vi "Pre Post Object File Path.vi"(6 "Post":string, 9 "Pre":string, 10 "Rename Library File Path":path) -> (1 "Post Object File Path":path, 2 "Pre Object File Path":path)   [LabVIEW 2025, in "_Rename.lvlib" / "_Rename.lvclass"]
uses:
  _Rename.lvclass
  _Rename.lvclass/_Rename.ctl
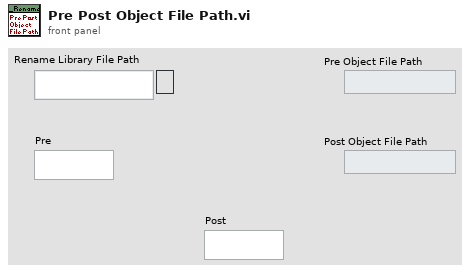
[diagram p1: front panel]
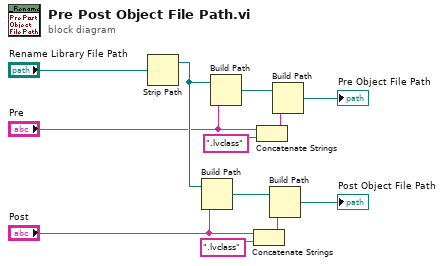
[diagram p0: block diagram]
diagram:
  n1 = Strip Path(path="Rename Library File Path") -> (stripped path=w5:path)  [unwired: 1 out]
  n2 = Build Path(base path=w5, name or relative path="Post") -> (appended path=w10:path)
  n3 = Build Path(base path=w5, name or relative path="Pre") -> (appended path=w7:path)
  n4 = Concatenate Strings("Post", ".lvclass" ("string")) -> (w12:string)
  n5 = Concatenate Strings("Pre", ".lvclass" ("string")) -> (w9:string)
  n6 = Build Path(base path=w10, name or relative path=w12) -> (appended path=→"Post Object File Path":path)
  n7 = Build Path(base path=w7, name or relative path=w9) -> (appended path=→"Pre Object File Path":path)
